vi "FromMatlabParam.vi"(4 "Allow Variant Values (f)":bool, 10 "Matlab Param Data":T1[](array[typedef]), 11 "Type (or value to update)":variant) -> (3 "Value":variant)   [LabVIEW 2017]
uses:
  Types/MatlabDataBundle.ctl
  Types/MatlabDataType.ctl
  Types/MatlabDataContainerType.ctl
panel:
  out "Conversion messages":string[](array[string])
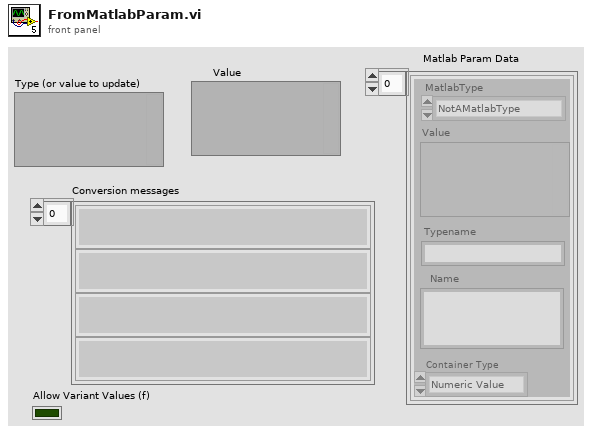
[diagram p1: front panel]
types:
  T1 = typedef "MatlabDataBundle.ctl" = cluster{"MatlabType":T2, "Value":variant, "Name":string, "Typename":string, "Container Type":T3}
  T2 = typedef "MatlabDataType.ctl" = enum16{"NotAMatlabType", "Real", "Complex", "String", "Boolean"}
  T3 = typedef "MatlabDataContainerType.ctl" = enum16{"Numeric Value", "Numeric Array", "Waveform"}
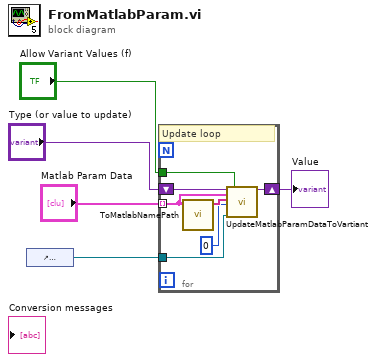
[diagram p0: block diagram]
diagram:
  n1 = control-ref of="Conversion messages"() -> (w2:refnum<vi>)
  n2 = for {
    tunnel: "Matlab Param Data" -> [w8] mode=indexing
    shift-right: [w10] -> w4
    shift-left: "Type (or value to update)" -> [w11]
    tunnel: w2 -> [w7]
    tunnel: "Allow Variant Values (f)" -> [w6]
    # "Update loop"
    n3 = call "ToMatlabNamePath.vi"("MatlabDataBundle"=w8) -> ("NamePath"=w12:string[])  [unwired: 10 in]
    n4 = call "UpdateMatlabParamDataToVartiant.vi"("Type (or value to update)"=w11, "MatlabDataBundle"=w8, "NamePath"=w12, "Namepath Index"=0 ("curNameIndex"), "Info collection refrence in"=w7, "Allow Variant Values (f)"=w6) -> ("Value"=w10:variant)  [unwired: 12 in, 1 out]
  }
  "Value" <- w4
